vi "User data.vi"(8 "Error In":errorcluster, 9 "Factory Name":string="EQD", 10 "Operator Name":string="ID-0") -> (0 "error out":errorcluster, 3 "refnum out":refnum<file>)   [LabVIEW 2018]
uses:
  LVU examples/SubVIs/Global textParse.vi
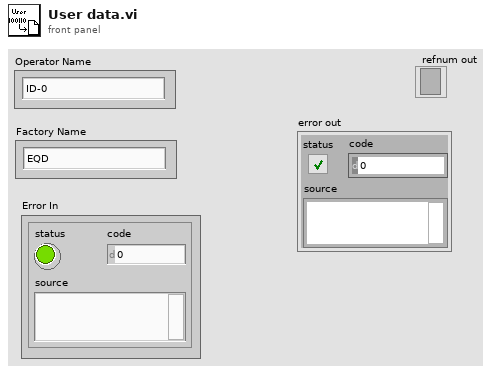
[diagram p1: front panel]
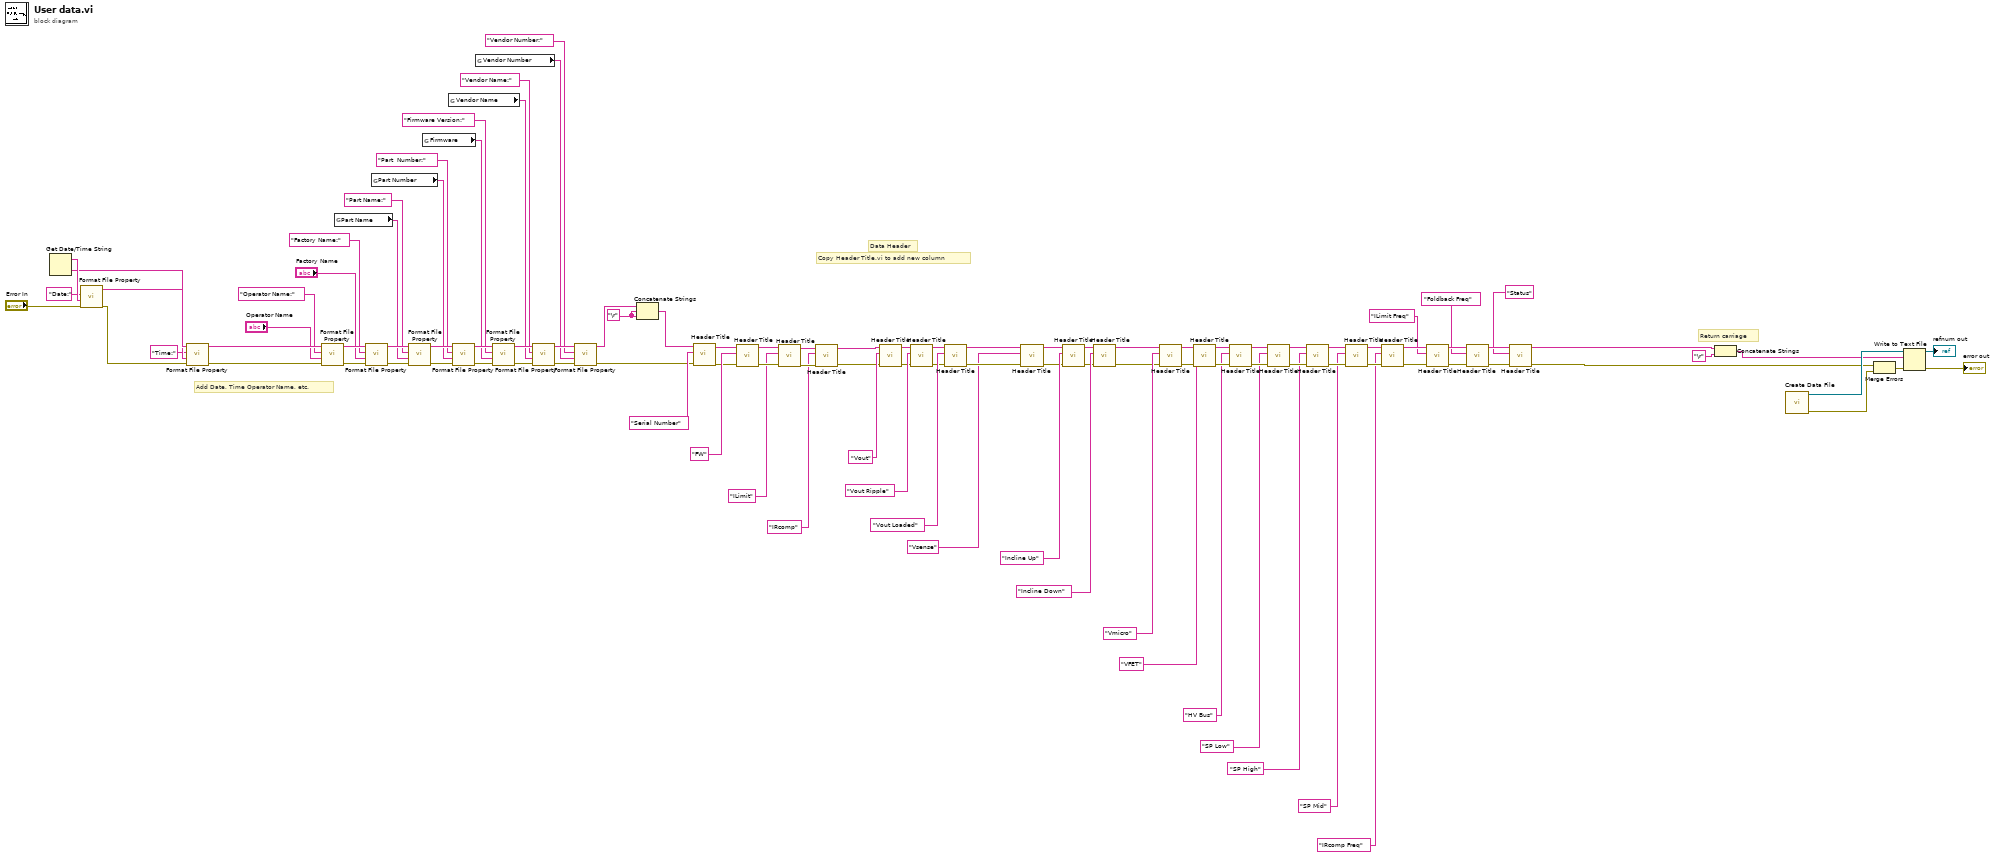
[diagram p0: block diagram]
diagram:
  w51 = "\r"
  # "Return carriage"
  # "Copy Header Title.vi to add new column"
  # "Data Header"
  # "Add Date, Time Operator Name, etc."
  n1 = Get Date/Time String() -> (date string=w95:string, time string=w83:string)  [unwired: 3 in]
  n2 = call "Format File Property.vi"("Error In"="Error In", "File Property Value"=w95, "File Property Name"="Date:") -> ("Error Out"=w91:errorcluster, "String out"=w94:string)  [unwired: 7 in]
  n3 = call "Format File Property.vi"("Error In"=w91, "File Property Value"=w83, "File Property Name"="Time:", "String in"=w94) -> ("Error Out"=w92:errorcluster, "String out"=w93:string)  [unwired: 6 in]
  n4 = call "Format File Property.vi"("Error In"=w92, "File Property Value"="Operator Name", "File Property Name"="Operator Name:", "String in"=w93) -> ("Error Out"=w90:errorcluster, "String out"=w89:string)  [unwired: 6 in]
  n5 = global read "Global textParse.vi" "Part Name"() -> (w79:string)
  n6 = call "Format File Property.vi"("Error In"=w90, "File Property Value"="Factory Name", "File Property Name"="Factory Name:", "String in"=w89) -> ("Error Out"=w81:errorcluster, "String out"=w82:string)  [unwired: 6 in]
  n7 = global read "Global textParse.vi" "Part Number"() -> (w97:string)
  n8 = call "Format File Property.vi"("Error In"=w81, "File Property Value"=w79, "File Property Name"="Part Name:", "String in"=w82) -> ("Error Out"=w80:errorcluster, "String out"=w103:string)  [unwired: 6 in]
  n9 = global read "Global textParse.vi" "Firmware"() -> (w100:string)
  n10 = global read "Global textParse.vi" "Vendor Name"() -> (w101:string)
  n11 = call "Format File Property.vi"("Error In"=w80, "File Property Value"=w97, "File Property Name"="Part  Number:", "String in"=w103) -> ("Error Out"=w96:errorcluster, "String out"=w104:string)  [unwired: 6 in]
  n12 = global read "Global textParse.vi" "Vendor Number"() -> (w102:string)
  n13 = call "Format File Property.vi"("Error In"=w96, "File Property Value"=w100, "File Property Name"="Firmware Version:", "String in"=w104) -> ("Error Out"=w98:errorcluster, "String out"=w105:string)  [unwired: 6 in]
  n14 = call "Format File Property.vi"("Error In"=w98, "File Property Value"=w101, "File Property Name"="Vendor Name:", "String in"=w105) -> ("Error Out"=w99:errorcluster, "String out"=w106:string)  [unwired: 6 in]
  n15 = call "Format File Property.vi"("Error In"=w99, "File Property Value"=w102, "File Property Name"="Vendor Number:", "String in"=w106) -> ("Error Out"=w55:errorcluster, "String out"=w53:string)  [unwired: 6 in]
  n16 = Concatenate Strings(w53, w51, w51) -> (w52:string)
  n17 = call "Header Title.vi"("Error In"=w55, "Header Title"="Serial Number" ("string"), "String in"=w52) -> ("Error Out"=w4:errorcluster, "String out"=w3:string)  [unwired: 7 in]
  n18 = call "Header Title.vi"("Error In"=w4, "Header Title"="FW", "String in"=w3) -> ("Error Out"=w11:errorcluster, "String out"=w10:string)  [unwired: 7 in]
  n19 = call "Header Title.vi"("Error In"=w11, "Header Title"="ILimit", "String in"=w10) -> ("Error Out"=w9:errorcluster, "String out"=w8:string)  [unwired: 7 in]
  n20 = call "Header Title.vi"("Error In"=w9, "Header Title"="IRcomp", "String in"=w8) -> ("Error Out"=w1:errorcluster, "String out"=w2:string)  [unwired: 7 in]
  n21 = call "Header Title.vi"("Error In"=w1, "Header Title"="Vout" ("string"), "String in"=w2) -> ("Error Out"=w56:errorcluster, "String out"=w60:string)  [unwired: 7 in]
  n22 = call "Header Title.vi"("Error In"=w56, "Header Title"="Vout Ripple" ("string"), "String in"=w60) -> ("Error Out"=w20:errorcluster, "String out"=w59:string)  [unwired: 7 in]
  n23 = call "Header Title.vi"("Error In"=w20, "Header Title"="Vout Loaded" ("string"), "String in"=w59) -> ("Error Out"=w16:errorcluster, "String out"=w19:string)  [unwired: 7 in]
  n24 = call "Header Title.vi"("Error In"=w16, "Header Title"="Vsense", "String in"=w19) -> ("Error Out"=w17:errorcluster, "String out"=w18:string)  [unwired: 7 in]
  n25 = call "Header Title.vi"("Error In"=w17, "Header Title"="Incline Up" ("Measured Data"), "String in"=w18) -> ("Error Out"=w15:errorcluster, "String out"=w58:string)  [unwired: 7 in]
  n26 = call "Header Title.vi"("Error In"=w15, "Header Title"="Incline Down" ("Measured Data"), "String in"=w58) -> ("Error Out"=w12:errorcluster, "String out"=w13:string)  [unwired: 7 in]
  n27 = call "Header Title.vi"("Error In"=w12, "Header Title"="Vmicro", "String in"=w13) -> ("Error Out"=w44:errorcluster, "String out"=w50:string)  [unwired: 7 in]
  n28 = call "Header Title.vi"("Error In"=w44, "Header Title"="VFET", "String in"=w50) -> ("Error Out"=w43:errorcluster, "String out"=w49:string)  [unwired: 7 in]
  n29 = call "Header Title.vi"("Error In"=w43, "Header Title"="HV Bus", "String in"=w49) -> ("Error Out"=w42:errorcluster, "String out"=w48:string)  [unwired: 7 in]
  n30 = call "Header Title.vi"("Error In"=w42, "Header Title"="SP Low", "String in"=w48) -> ("Error Out"=w41:errorcluster, "String out"=w47:string)  [unwired: 7 in]
  n31 = call "Header Title.vi"("Error In"=w41, "Header Title"="SP High", "String in"=w47) -> ("Error Out"=w40:errorcluster, "String out"=w46:string)  [unwired: 7 in]
  n32 = call "Header Title.vi"("Error In"=w40, "Header Title"="SP Mid", "String in"=w46) -> ("Error Out"=w39:errorcluster, "String out"=w45:string)  [unwired: 7 in]
  n33 = call "Header Title.vi"("Error In"=w39, "Header Title"="IRcomp Freq", "String in"=w45) -> ("Error Out"=w27:errorcluster, "String out"=w31:string)  [unwired: 7 in]
  n34 = call "Header Title.vi"("Error In"=w27, "Header Title"="ILimit Freq", "String in"=w31) -> ("Error Out"=w26:errorcluster, "String out"=w30:string)  [unwired: 7 in]
  n35 = call "Header Title.vi"("Error In"=w26, "Header Title"="Foldback Freq", "String in"=w30) -> ("Error Out"=w25:errorcluster, "String out"=w29:string)  [unwired: 7 in]
  n36 = call "Header Title.vi"("Error In"=w25, "Header Title"="Status", "String in"=w29) -> ("Error Out"=w24:errorcluster, "String out"=w28:string)  [unwired: 7 in]
  n37 = Concatenate Strings(w28, "\r") -> (w54:string)
  n38 = call "Create Data File.vi"() -> ("Error Out"=w84:errorcluster, "File Refnum"=w86:refnum<file>)  [unwired: 10 in]
  n39 = Merge Errors(w24, w84) -> (w85:errorcluster)
  n40 = Write to Text File(file (use dialog)=w86, text=w54, error in=w85) -> (refnum out=→"refnum out":refnum<file>, error out=→"error out":errorcluster)  [unwired: 1 in, 1 out]
